vi "Fix Buttonn Array Size.vi"(1 "Number of Buttons":i32, 2 "Button States In":refnum<class "Button.lvclass">[](array[class])) -> (0 "Button States Out":refnum<class "Button.lvclass">[](array[class]))   [LabVIEW 2012, in "Toolbar.xctl"]
doc: "Expands the array of buttons to the required length if necessary."
uses:
  Toolbar.xctl
  Button_Class/Button.lvclass
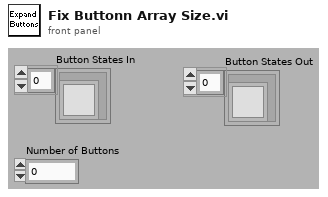
[diagram p1: front panel]
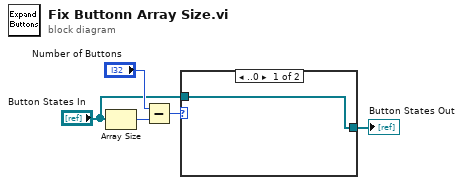
[diagram p0: block diagram]
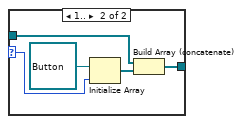
[diagram p2: hidden frame]
diagram:
  n1 = Array Size(array="Button States In") -> (size(s)=w1:i32)
  n2 = Subtract(x="Number of Buttons", y=w1) -> (x-y=w4:i32)
  n3 = case shown="..0" w4 {
    selector: w4 -> [_ w11]
    tunnel: "Button States In" -> [w6 w8]
    tunnel: [w6 w7] -> w5
    frame ..0 {
    }
    frame 1.. {
      n4 = Initialize Array(refnum<class "Button.lvclass"> refnum ("Button.lvclass"), w11) -> (w9:refnum<class "Button.lvclass">[])
      n5 = Build Array (concatenate)(w8, w9) -> (w7:refnum<class "Button.lvclass">[])
    }
  }
  "Button States Out" <- w5
